vi "AddOption_Legend.vi"(0 "reference in":refnum<class "HTMLPlot.lvclass">, 2 "OptionsIn":string[](array[string]), 5 "error in (no error)":errorcluster) -> (14 "reference out":refnum<class "HTMLPlot.lvclass">, 16 "OptionsOut":string[](array[string]), 19 "error out":errorcluster)   [LabVIEW 2019, in "HTMLPlot.lvclass"]
uses:
  HTMLPlot.lvclass
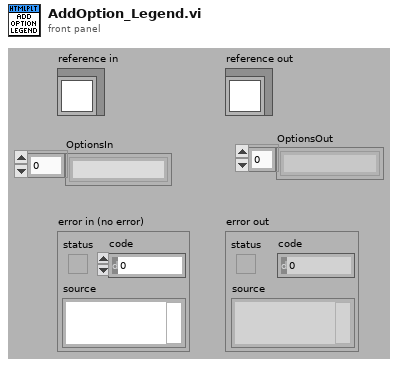
[diagram p1: front panel]
types:
  T1 = typedef "HTMLPlot.lvclass/ObjectAttributes.ctl" = cluster{"Attribute1":dbl, "GraphContainer":refnum<k7>, "ChartScriptFile":string, "UtilScriptFile(demoData)":string, "BaseHTML":string, "GenericProperties":cluster{"PlotType":T2, "PlotTitle":string, "XLabel":string, "YLabel":string, "ShowToolTip":bool}, "LegendProperties":cluster{"Show":bool, "Position":T3}, "BarPlot":cluster{"Dataset":dbl[][], "DatasetLabels":string[], "XLabels":string[], "PlotColours":u32[], "Stacked":bool}, "PiePlot":cluster{"Dataset":dbl[][], "DatasetLabels":string[], "PlotColours":u32[], "DoughnutStyle":bool, "PlotLabels":string[]}, "connection ID":refnum<k5>, "PortID":u64}
  T2 = typedef "HTMLPlot.lvclass/PlotType.ctl" = enum16{"bar", "line", "pie"}
  T3 = typedef "HTMLPlot.lvclass/LegendPosition.ctl" = enum16{"top", "right", "left", "bottom"}
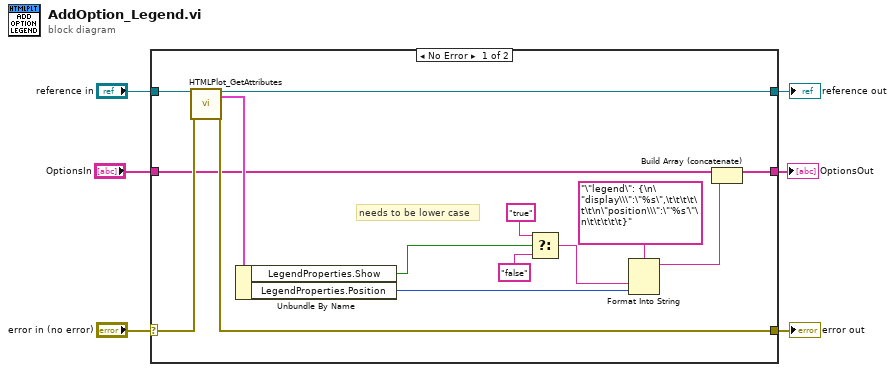
[diagram p0: block diagram]
diagram:
  n1 = case shown="No Error" "error in (no error)" {
    selector: "error in (no error)" -> [w20 w23]
    tunnel: [w18 w23] -> w5
    tunnel: [w16 w22] -> w3
    tunnel: "reference in" -> [w17 w22]
    tunnel: "OptionsIn" -> [w15 w21]
    tunnel: [w14 w21] -> w1
    frame No Error {
      # "needs to be lower case"
      n2 = call "HTMLPlot_GetAttributes.vi"("reference in"=w17, "error in (no error)"=w20) -> ("reference out"=w16:refnum<class "HTMLPlot.lvclass">, "Data"=w19:T1, "error out"=w18:errorcluster)  [unwired: 14 in, 1 out]
      n3 = Unbundle By Name(w19) -> ("LegendProperties.Show"=w8:bool, "LegendProperties.Position"=w13:T3)
      n4 = Select(t="true", s=w8, f="false") -> (s? t:f=w7:string)
      n5 = Format Into String(format string="\"legend\": {\n\"display\\\":\"%s\",\t\t\t\t\t\t\n\"position\\\":\"'%s'\"\n\t\t\t\t\t}", w7, w13) -> (resulting string=w11:string)  [unwired: 2 in, 1 out]
      n6 = Build Array (concatenate)(w15, w11) -> (w14:string[])
    }
    frame Error {
    }
  }
  "error out" <- w5
  "reference out" <- w3
  "OptionsOut" <- w1
